vi "Read Coils.vi"(8 "error in (no error)":errorcluster, 9 "number of coils":i32=1, 10 "address":i32, 11 "modbus in":refnum<class "libmodbus.lvclass">) -> (0 "error out":errorcluster, 2 "coils":bool[](array[boolean]), 3 "modbus out":refnum<class "libmodbus.lvclass">)   [LabVIEW 2017, in "libmodbus.lvlib" / "libmodbus.lvclass"]
doc: "Reads multiple coils."
uses:
  libmodbus.lvclass
  libmodbus.lvclass/libmodbus.ctl
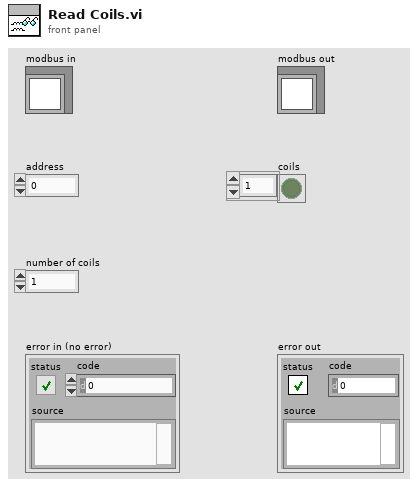
[diagram p1: front panel]
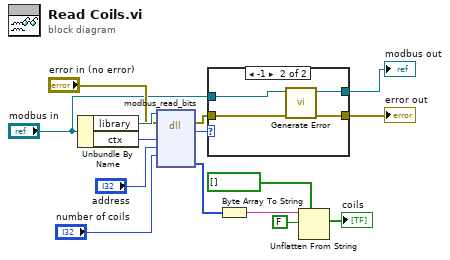
[diagram p0: block diagram]
diagram:
  n1 = Unbundle By Name("modbus in") -> ("library"=w14:path, "ctx"=w15:i64)
  n2 = dll-call lib="?" fn="modbus_read_bits"(path in=w14, error in="error in (no error)", "ctx"=w15, "addr"="address", "nb"="number of coils") -> (error out=w10:errorcluster, "int"=w12:i32, "dest"=w4:u8[])  [unwired: 5 in, 1 out]
  n3 = case shown="-1" w12 {
    tunnel: [w17 w20] -> w11
    tunnel: w10 -> [w17 w21]
    tunnel: "modbus in" -> [w16 w19]
    tunnel: [w16 w18] -> w8
    frame Default {
    }
    frame -1 {
      n4 = call "Generate Error.vi"("error in (no error)"=w21, "modbus in"=w19) -> ("error out"=w20:errorcluster, "modbus out"=w18:refnum<class "libmodbus.lvclass">)  [unwired: 8 in]
    }
  }
  "modbus out" <- w8
  "error out" <- w11
  n5 = Byte Array To String(unsigned byte array=w4) -> (string=w3:string)
  n6 = Unflatten From String(type=bool[] [] ("data includes array or string size? (T)"), binary string=w3, data includes array or string size? (T)=FALSE) -> (value=→"coils":bool[])  [unwired: 2 in, 2 out]
